vi "create sorted list.vi"(11 "list":string[](array[string])) -> (3 "sorted list":T1)   [LabVIEW 2013, in "tag bus.lvlib" / "binary search.lvlib"]
doc: "Takes a list of strings and converts them into a sorted list, preserving the original indices. This can be reversed by reorder list.vi."
uses:
  binary search.lvlib
  sorted list.ctl
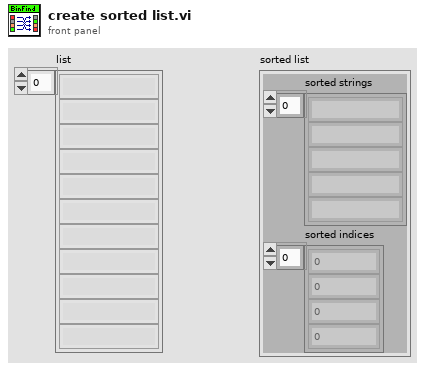
[diagram p1: front panel]
types:
  T1 = typedef "tag bus.lvlib/binary search.lvlib/sorted list.ctl" = cluster{"sorted strings":string[], "sorted indices":i32[]}
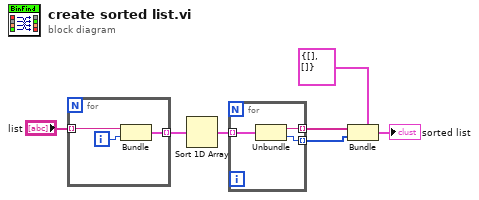
[diagram p0: block diagram]
diagram:
  n1 = for {
    tunnel: "list" -> [w8] mode=indexing
    tunnel: [w10] -> w6 mode=indexing
    i -> [w9]
    n2 = Bundle("String"=w8, w9) -> (w10:cluster{"String":string, i32})  [unwired: 1 in]
  }
  n3 = Sort 1D Array(array=w6) -> (sorted array=w5:cluster{"String":string, i32}[])
  n4 = for {
    tunnel: w5 -> [w13] mode=indexing
    tunnel: [w12] -> w2 mode=indexing
    tunnel: [w11] -> w1 mode=indexing
    n5 = Unbundle(w13) -> ("String"=w12:string, w11:i32)
  }
  n6 = Bundle(cluster=T1 {"sorted strings"=[], "sorted indices"=[]} ("sorted list"), "sorted strings"=w2, "sorted indices"=w1) -> (→"sorted list":T1)
